vi "Resolve Group Conflicts.vi"(8 "error in (no error)":errorcluster, 9 "Current Group Number (0)":i32, 10 "Group Name in":string, 11 "TDMS Log File in":refnum<class "TDMS Log File.lvclass">) -> (0 "error out":errorcluster, 1 "Group Number":i32, 2 "Group Name out":string, 3 "TDMS Log File out":refnum<class "TDMS Log File.lvclass">)   [LabVIEW 2015, in "TDMS Log File.lvclass"]
uses:
  TDMS Log File.lvclass
  TDMS Log File.lvclass/TDMS Log File.ctl
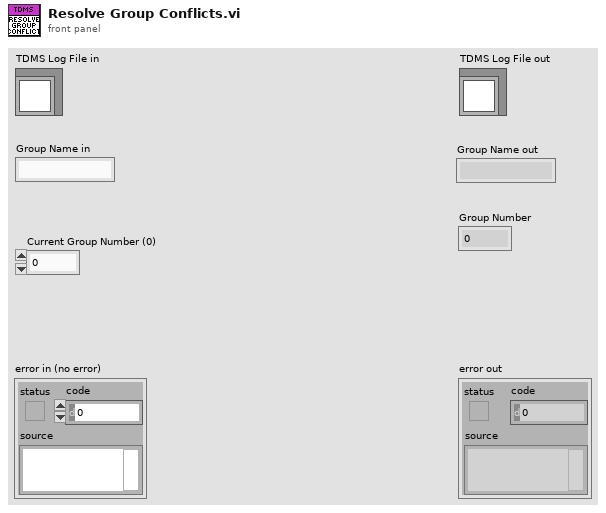
[diagram p1: front panel]
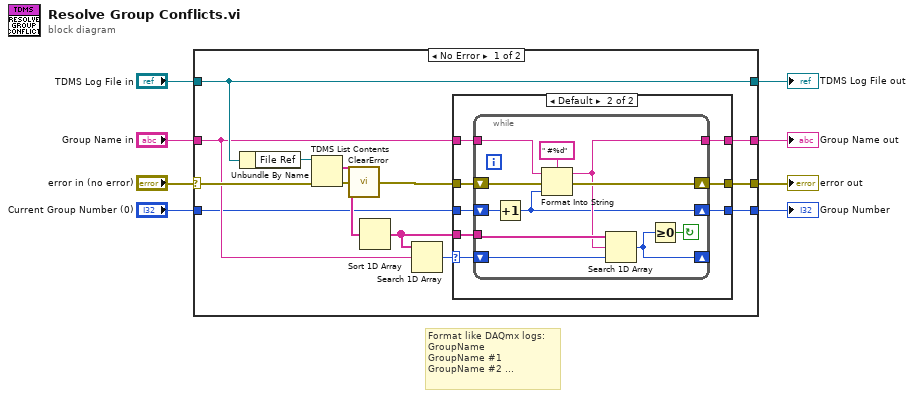
[diagram p0: block diagram]
diagram:
  # "Format like DAQmx logs:\nGroupName\nGroupName #1\nGroupName #2 ..."
  n1 = case shown="No Error" "error in (no error)" {
    selector: "error in (no error)" -> [w19 w46]
    tunnel: [w14 w46] -> w7
    tunnel: [w21 w45] -> w5
    tunnel: "TDMS Log File in" -> [w21 w45]
    tunnel: "Group Name in" -> [w17 w44]
    tunnel: [w16 w44] -> w3
    tunnel: "Current Group Number (0)" -> [w11 w43]
    tunnel: [w10 w43] -> w1
    frame No Error {
      n2 = Unbundle By Name(w21) -> ("File Ref"=w20:refnum<k34>)
      n3 = TDMS List Contents(4:w19, 7:w20) -> (0:w9:errorcluster, 2:w13:string[])  [unwired: 1 in, 2 out]
      n4 = call <vilib>:"ClearError.vi"("error in (no error)"=w9) -> ("error out"=w15:errorcluster)
      n5 = Sort 1D Array(array=w13) -> (sorted array=w12:string[])
      n6 = Search 1D Array(1D array=w12, element=w17) -> (index of element=w18:i32)  [unwired: 1 in]
      n7 = case shown="Default" w18 {
        selector: w18 -> [_ w26]
        tunnel: w17 -> [w23 w29]
        tunnel: [w23 w28] -> w16
        tunnel: w15 -> [w22 w31]
        tunnel: w12 -> [_ w30]
        tunnel: [w22 w27] -> w14
        tunnel: w11 -> [_ w25]
        tunnel: [_ w24] -> w10
        frame -1 {
          # "Group does not\ncurrently exist in file.\nUse as-is."
        }
        frame Default {
          n8 = while {
            shift-right: [w37] -> w27
            shift-left: w31 -> [w42]
            tunnel: w30 -> [w39]
            tunnel: w29 -> [w40]
            tunnel: [w36] -> w28
            shift-right: [w34] -> _
            shift-left: w26 -> [w35]
            shift-right: [w32] -> w24
            shift-left: w25 -> [w33]
            stop <- w38 continue-if-true
            n9 = Increment(x=w33) -> (x+1=w32:i32)
            n10 = Format Into String(format string=" #%d", initial string=w40, error in=w42, w32) -> (resulting string=w36:string, error out=w37:errorcluster)
            n11 = Search 1D Array(1D array=w39, element=w36, start index (0)=w35) -> (index of element=w34:i32)
            n12 = Greater Or Equal To 0?(x=w34) -> (x >= 0?=w38:bool)
          }
        }
      }
    }
    frame Error {
    }
  }
  "error out" <- w7
  "TDMS Log File out" <- w5
  "Group Name out" <- w3
  "Group Number" <- w1
